vi "lv_mysql_conn_close.vi"(8 "error in (no error)":errorcluster, 11 "connection ID":refnum<k5>) -> (0 "error out":errorcluster)   [LabVIEW 2020]
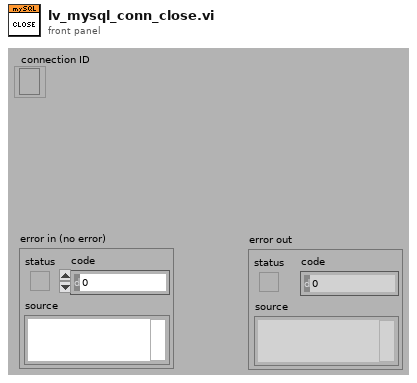
[diagram p1: front panel]
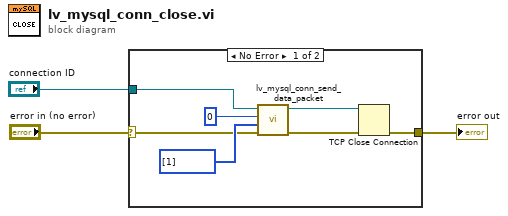
[diagram p0: block diagram]
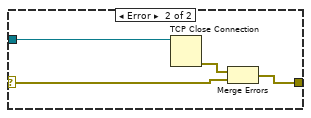
[diagram p2: hidden frame]
diagram:
  n1 = case shown="No Error" "error in (no error)" {
    selector: "error in (no error)" -> [w4 w12]
    tunnel: "connection ID" -> [w10 w14]
    tunnel: [w5 w11] -> w2
    frame No Error {
      n2 = call "lv_mysql_conn_send_data_packet.vi"("error in"=w4, "TCP/IP Data"=u8[] [1], "Packet #"=u8 0, "connection ID"=w10) -> ("error out"=w6:errorcluster, "connection ID out"=w7:refnum<k5>)  [unwired: 6 in]
      n3 = TCP Close Connection(connection ID=w7, error in (no error)=w6) -> (error out=w5:errorcluster)  [unwired: 1 in, 1 out]
    }
    frame Error {
      n4 = TCP Close Connection(connection ID=w14) -> (error out=w13:errorcluster)  [unwired: 2 in, 1 out]
      n5 = Merge Errors(w13, w12) -> (w11:errorcluster)
    }
  }
  "error out" <- w2
